vi "get_Network.vi"(0 "Host_Reference":refnum<class "HGF_Reference.lvclass">, 2 "timeout in ms (-1)":i32=-1, 5 "error in (no error)":errorcluster) -> (14 "dup Host_Reference":refnum<class "HGF_Reference.lvclass">, 16 "Network":T1, 19 "error out":errorcluster)   [LabVIEW 2009, in "MoAgSy.lvlib" / "MoAgSy_Host.lvclass"]
doc: "<B>public</B> VI returns network events from referenced Host.\nNetwork Events are used for the systems communication.\n\nF.Berck@gsi.de\nGSI Darmstadt 2009"
uses:
  MoAgSy_Host.lvclass
  HGF_BaseClasses/HGF_Reference/HGF_Reference.lvclass
  HGF_BaseClasses/HGF_Event/HGF_Event.lvclass
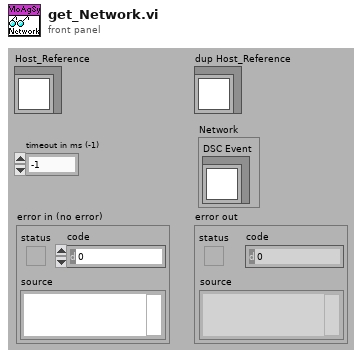
[diagram p1: front panel]
types:
  T1 = cluster{"DSC Event":refnum<class "HGF_Event.lvclass">}
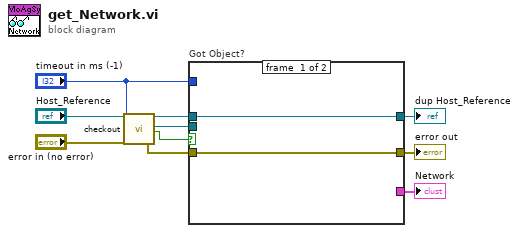
[diagram p0: block diagram]
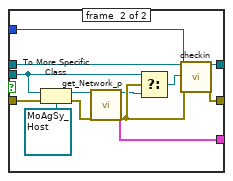
[diagram p2: hidden frame]
diagram:
  n1 = call "checkout.vi"("HGF_Reference"="Host_Reference", "timeout in ms (-1)"="timeout in ms (-1)", "error in (no error)"="error in (no error)") -> ("dup HGF_Reference"=w5:refnum<class "HGF_Reference.lvclass">, "Object"=w8:refnum<class>, "got object?"=w6:bool, "error out"=w9:errorcluster)  [unwired: 13 out]
  n2 = case "Got Object?" shown="True" w6 {
    tunnel: w9 -> [w11 w25]
    tunnel: w8 -> [_ w16]
    tunnel: w5 -> [w12 w23]
    tunnel: [w12 w22] -> w4
    tunnel: "timeout in ms (-1)" -> [_ w21]
    tunnel: [w11 w20] -> w2
    tunnel: [_ w18] -> w1
    frame #0 {
    }
    frame #1 {
      n3 = To More Specific Class(target class=refnum<class "MoAgSy_Host.lvclass"> refnum ("MoAgSy.lvlib:MoAgSy_Host.lvclass"), reference=w16, error in=w25) -> (specific class reference=w19:refnum<class "MoAgSy_Host.lvclass">, error out=w17:errorcluster)
      n4 = call "get_Network_p.vi"("MoAgSy_Host"=w19, "error in (no error)"=w17) -> ("dup MoAgSy_Host"=w13:refnum<class "MoAgSy_Host.lvclass">, "Network Events"=w18:T1, "error out"=w14:errorcluster)  [unwired: 15 out]
      n5 = Select(t=w16, s=w14, f=w13) -> (s? t:f=w15:refnum<class>)
      n6 = call "checkin.vi"("HGF_Reference"=w23, "Object"=w15, "timeout /ms (-1)"=w21, "error in (no error)"=w14) -> ("dup HGF_Reference"=w22:refnum<class "HGF_Reference.lvclass">, "error out"=w20:errorcluster)  [unwired: 14 out]
    }
  }
  "dup Host_Reference" <- w4
  "error out" <- w2
  "Network" <- w1
